vi "变体数组转换模板-（不可运行）.vi"   [LabVIEW 2013]
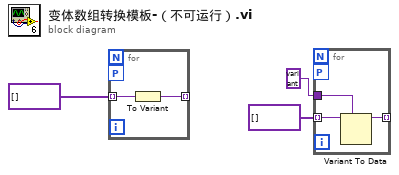
[diagram p0: block diagram]
diagram:
  n1 = for {
    workers-P: _ -> [_]
    tunnel: variant[] [] -> [w5] mode=indexing
    tunnel: [w4] -> _ mode=indexing
    n2 = To Variant(anything=w5) -> (Variant=w4:variant)
  }
  n3 = for {
    workers-P: _ -> [_]
    tunnel: variant[] [] -> [w8] mode=indexing
    tunnel: variant ("变体") -> [w7]
    tunnel: [w6] -> _ mode=indexing
    n4 = Variant To Data(type=w7, Variant=w8) -> (data=w6:variant)  [unwired: 1 in, 1 out]
  }
